vi "Laser Fine Cutting.vi"(0 "configuration file path":path=path "C:/Users/admin/OneDrive/文档/Inlafa.CCV254.MES/System/All Config.ini" caption="配置文件的路径", 1 "fine cutting msic":T1) -> ()   [LabVIEW 2018]
uses:
  Ctl.xio/fine cutting msic ctl.ctl
  SubVIS.xio/DataSocket/DataSocket_Tags.ctl
  Ctl.xio/part type.ctl
  SubVIS.xio/Creat Write List VI's/DefCtrl/Station.ctl
  SubVIS.xio/DataSocket/Write PLC Vars/Write String Var in.vi
  <vilib>/Utility/file.llb/Read From Spreadsheet File (string).vi
  SubVIS.xio/DataSocket/Write PLC Vars/Write Bool Var in.vi
  SubVIS.xio/DataSocket/Read PLC Vars/Read String Var.vi
  SubVIS.xio/DataSocket/Write PLC Vars/Write Dbl Var in.vi
  SubVIS.xio/DataSocket/Read PLC Vars/Read Bool Var.vi
panel:
  in  "SQL information":string
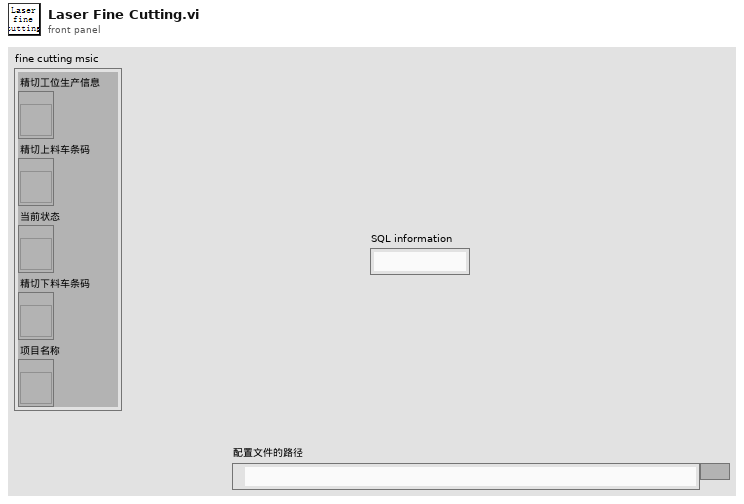
[diagram p1: front panel]
types:
  T1 = cluster{"精切工位生产信息":refnum<vi>, "精切上料车条码":refnum<vi>, "当前状态":refnum<vi>, "精切下料车条码":refnum<vi>, "项目名称":refnum<vi>}
  T2 = typedef "Station.ctl" = enum16{"粗切工位", "热处理工位", "精切工位", "PDF焊接工位", "打凹点预载力工位", "收卷工位", "EOL工位"}
  T3 = typedef "fine cutting msic ctl.ctl" = cluster{"configuration file path":path, "DsOut":T4[], "incar information A":cluster{"incar code":string, "incar No":string, "incar plate No":string, "cut time":string}, "pallet A.No_output":i32, "SQL information":string, "Database":string[], "Serial number":i32, "database path":path, "fine cutting msic":cluster{"production info":refnum<vi>, "incar code":refnum<vi>, "status":refnum<vi>, "outcar code":refnum<vi>, "part type":refnum<vi>}, "part type":T5, "scanner1 coms":string, "scanner2 coms":string, "scanner1 resource name out":refnum<visa-resource-name>, "scanner2 resource name out":refnum<visa-resource-name>, "incar code A":string, "outcar code":string, "outcar information":cluster{"outcar code":string, "outcar No":string, "outcar plate No":string, "cut time":string}, "scanner1 ip ID":refnum<k5>, "scanner2 ip ID":refnum<k5>, "Number of scans":i32, "Cut file":string, "Process code":string, "second?":bool, "incar code B":string, "incar information B":cluster{"incar code":string, "incar No":string, "incar plate No":string, "cut time":string}, "pallet B.No_output":i32}
  T4 = typedef "DataSocket_Tags.ctl" = cluster{"Ds ID":refnum<k13>, "Tag":string}
  T5 = typedef "part type.ctl" = cluster{"Part type":string, "Material code":string, "Part number":string, "Supplier code":string, "Line code":string, "Customer code":string, "Color code":string, "Upper limit":i32, "Temperature":string, "Tot time":string, "EOL stations":string}
  T6 = cluster{"incar code":string, "incar No":string, "incar plate No":string, "cut time":string}
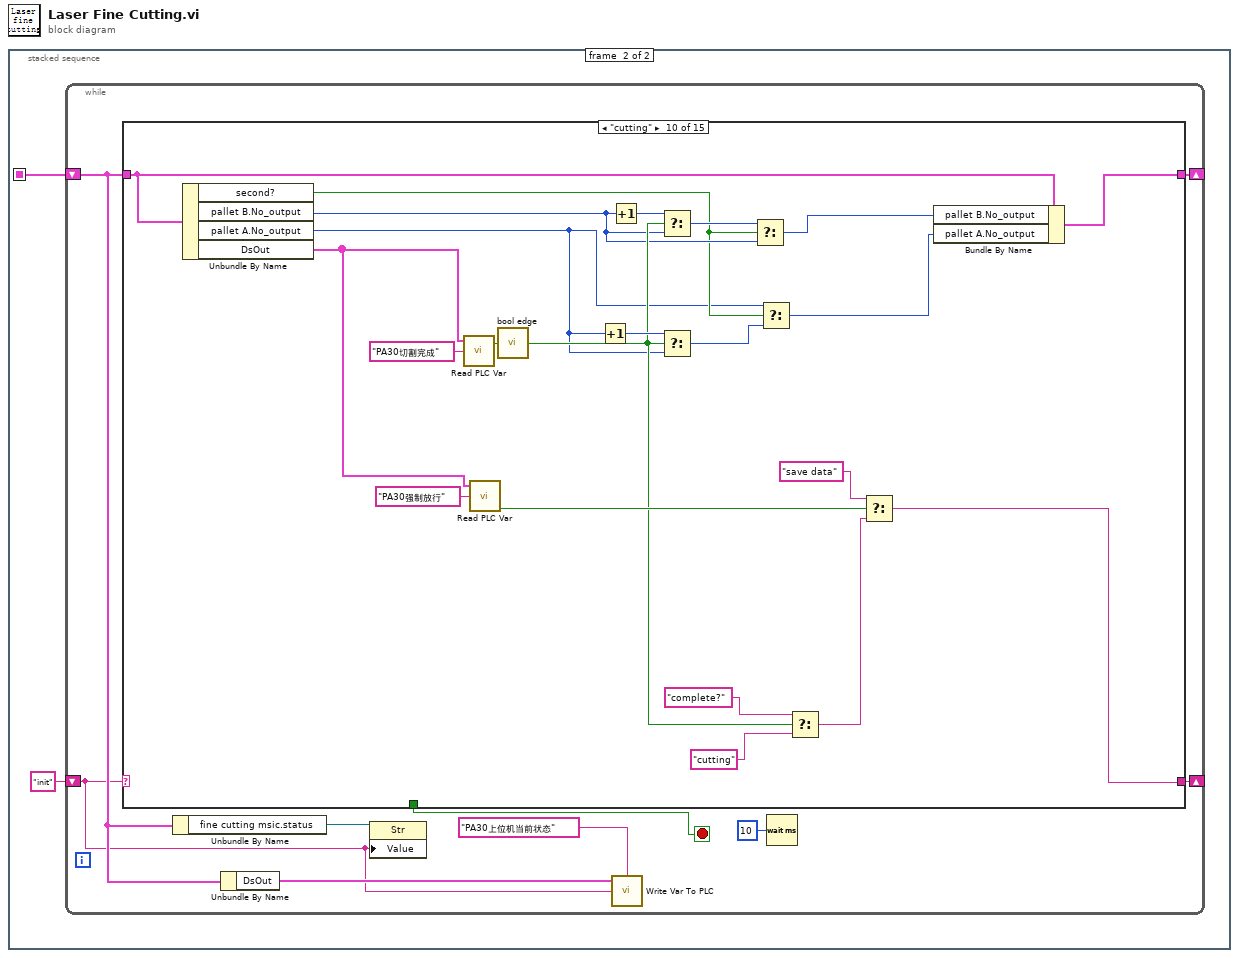
[diagram p0: block diagram]
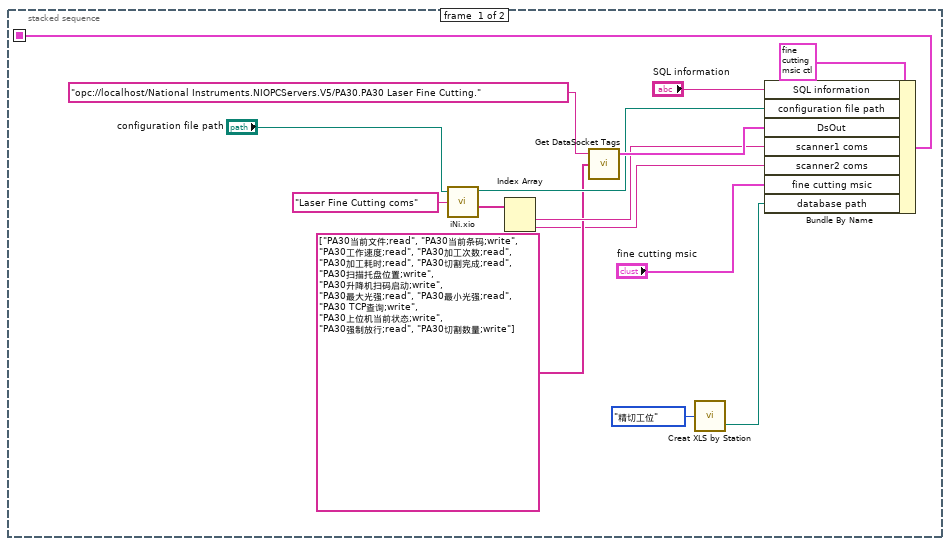
[diagram p2: hidden frame]
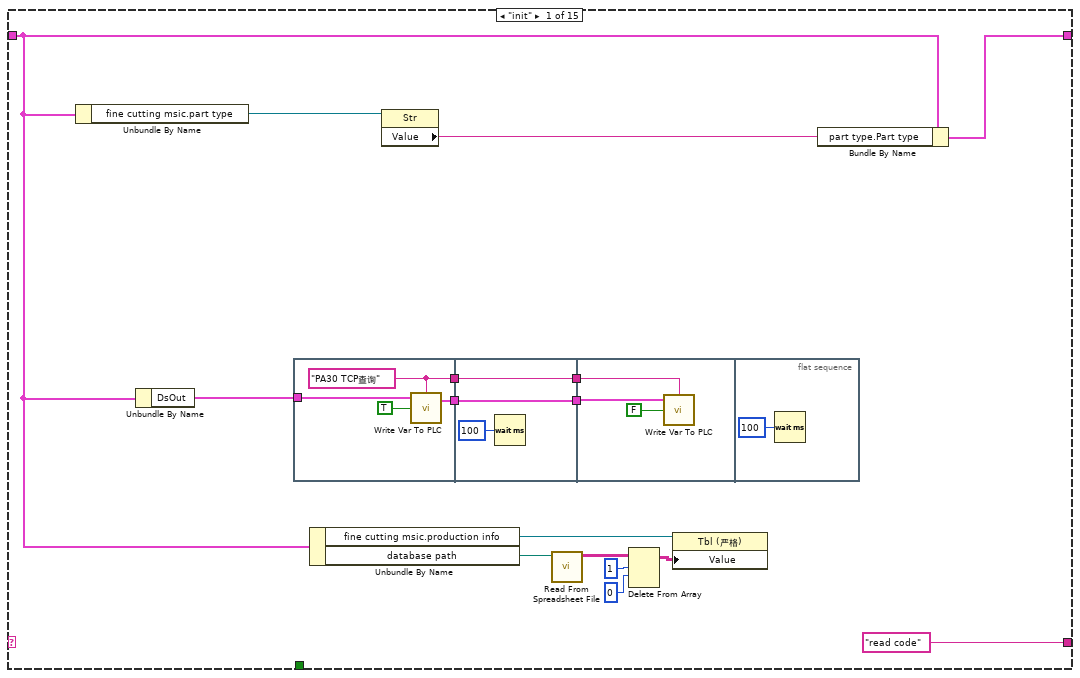
[diagram p3: hidden frame]
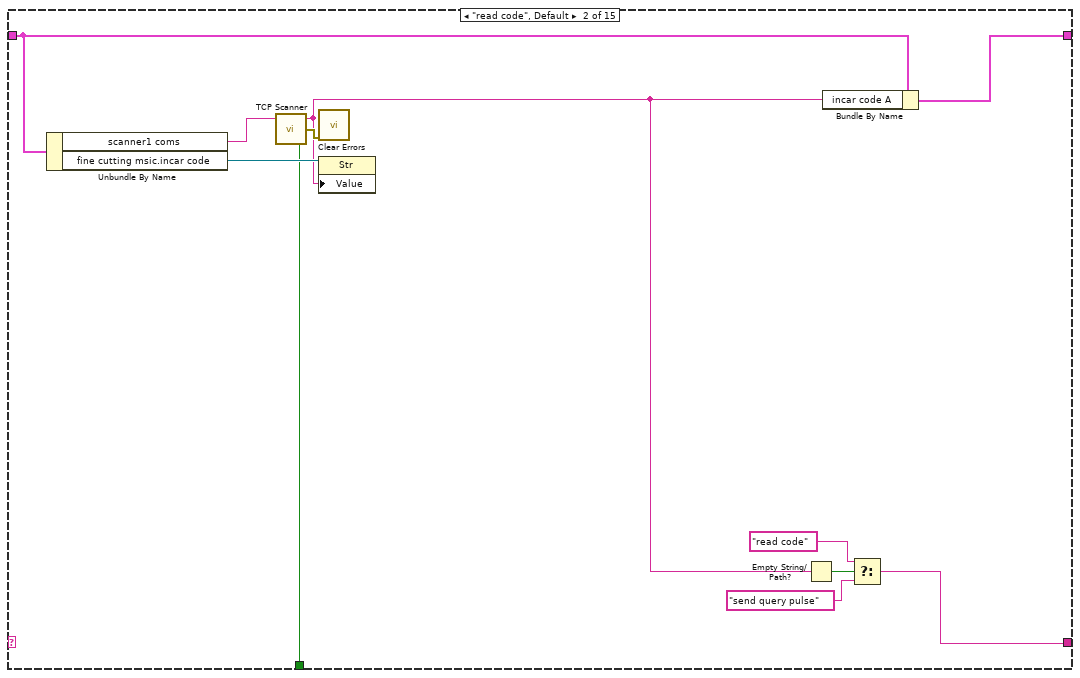
[diagram p4: hidden frame]
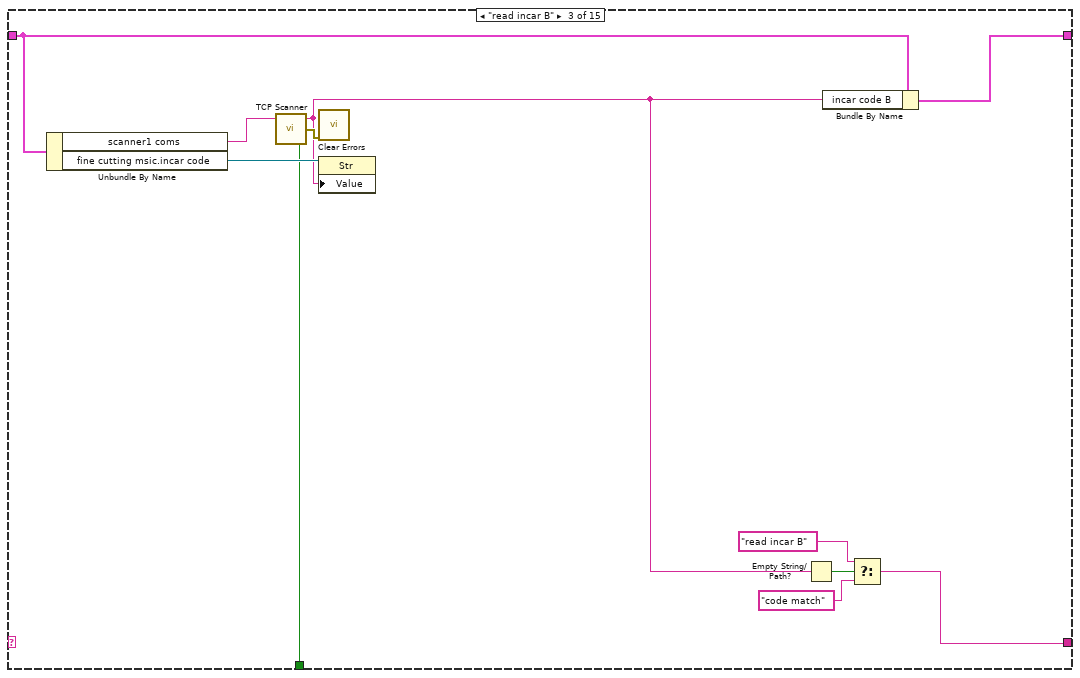
[diagram p5: hidden frame]
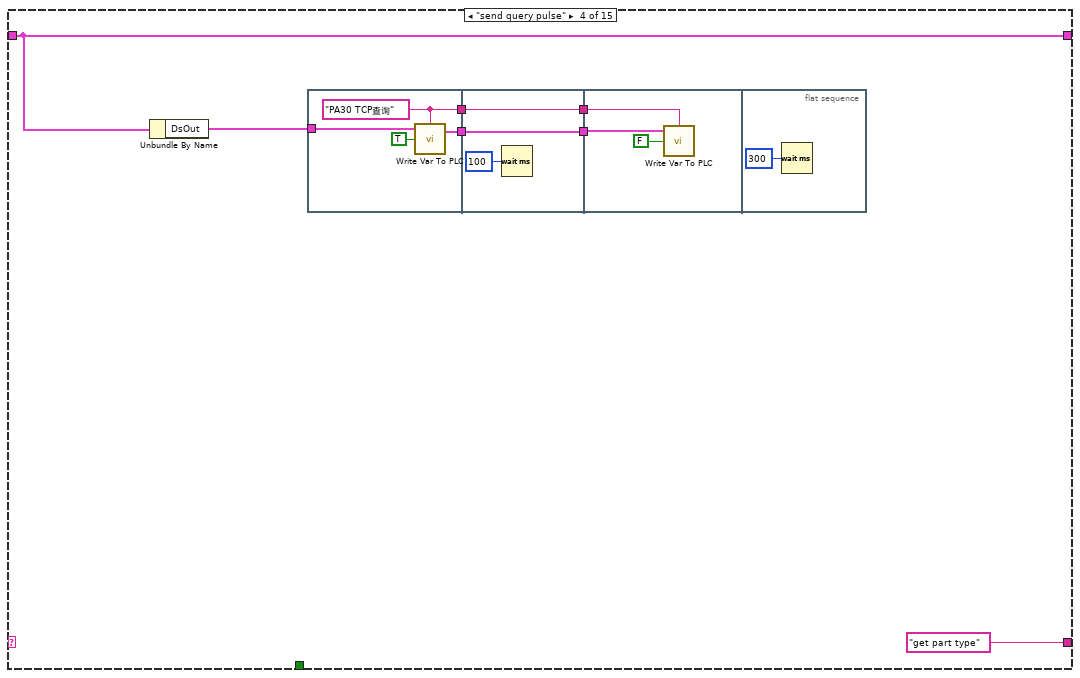
[diagram p6: hidden frame]
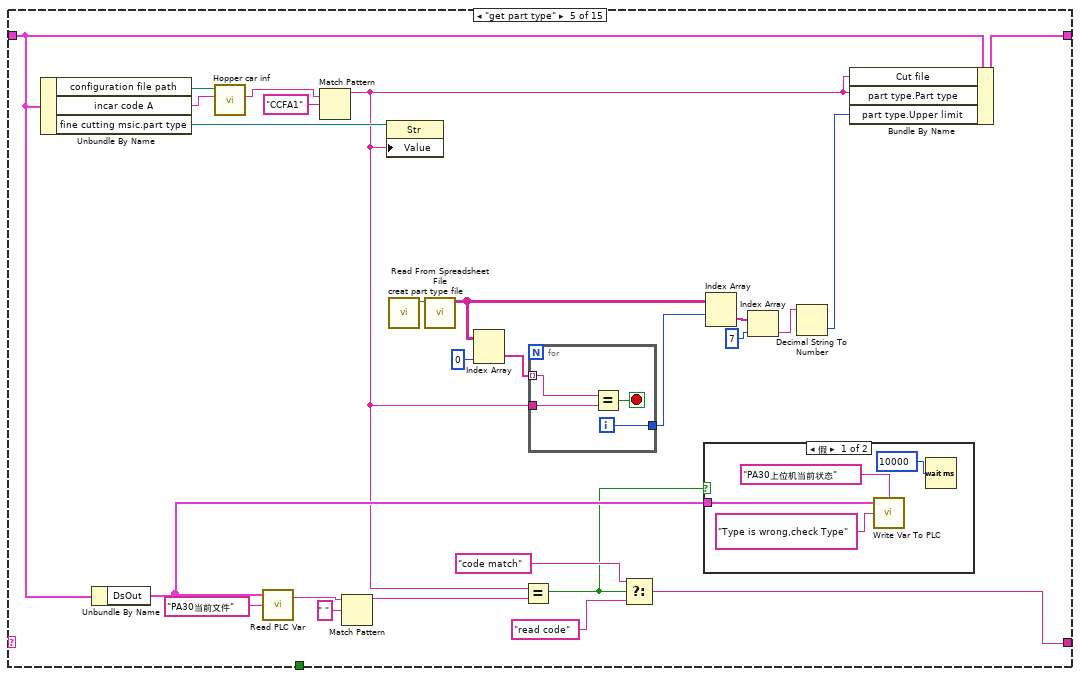
[diagram p7: hidden frame]
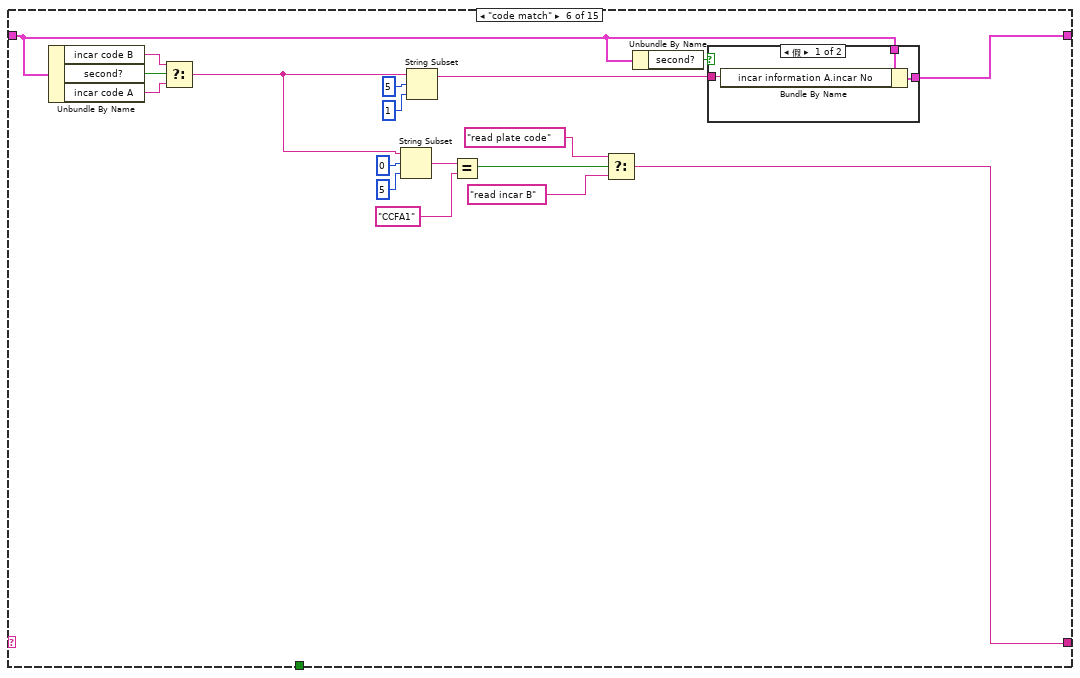
[diagram p9: hidden frame]
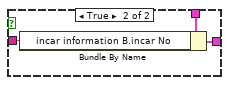
[diagram p10: hidden frame]
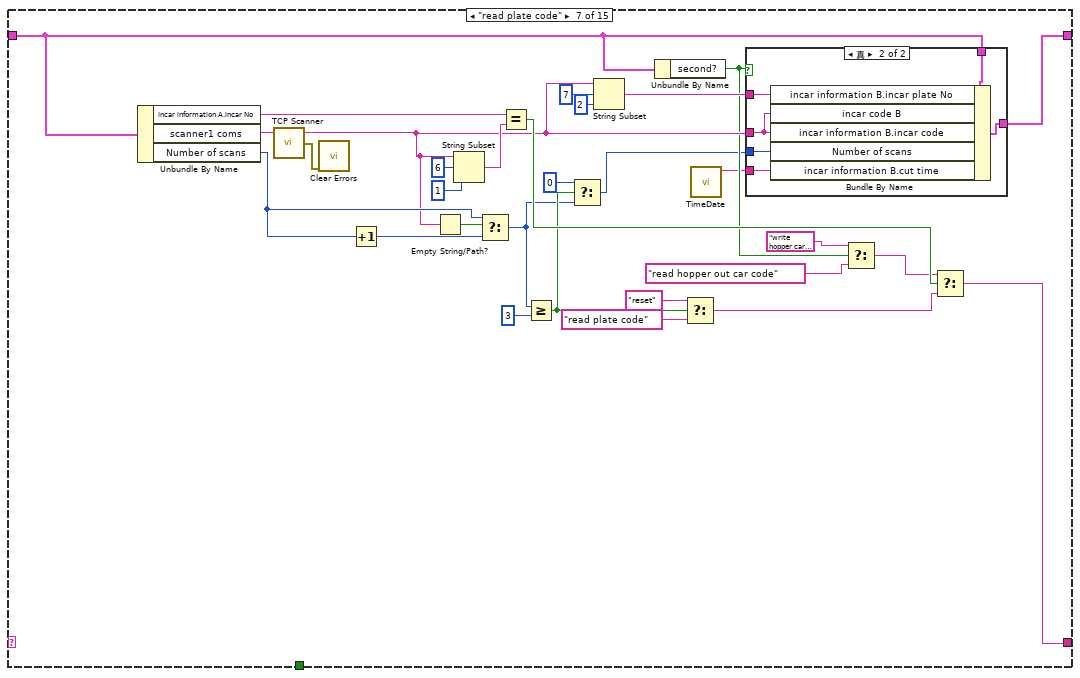
[diagram p11: hidden frame]
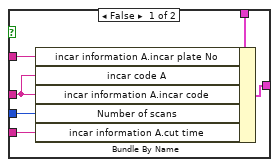
[diagram p12: hidden frame]
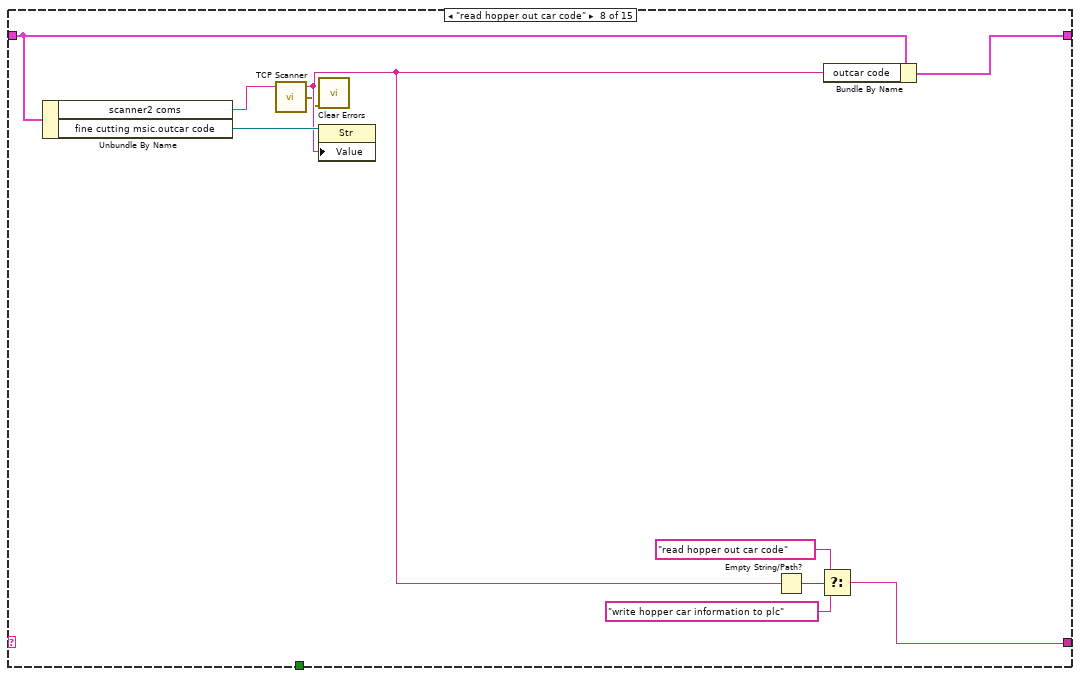
[diagram p13: hidden frame]
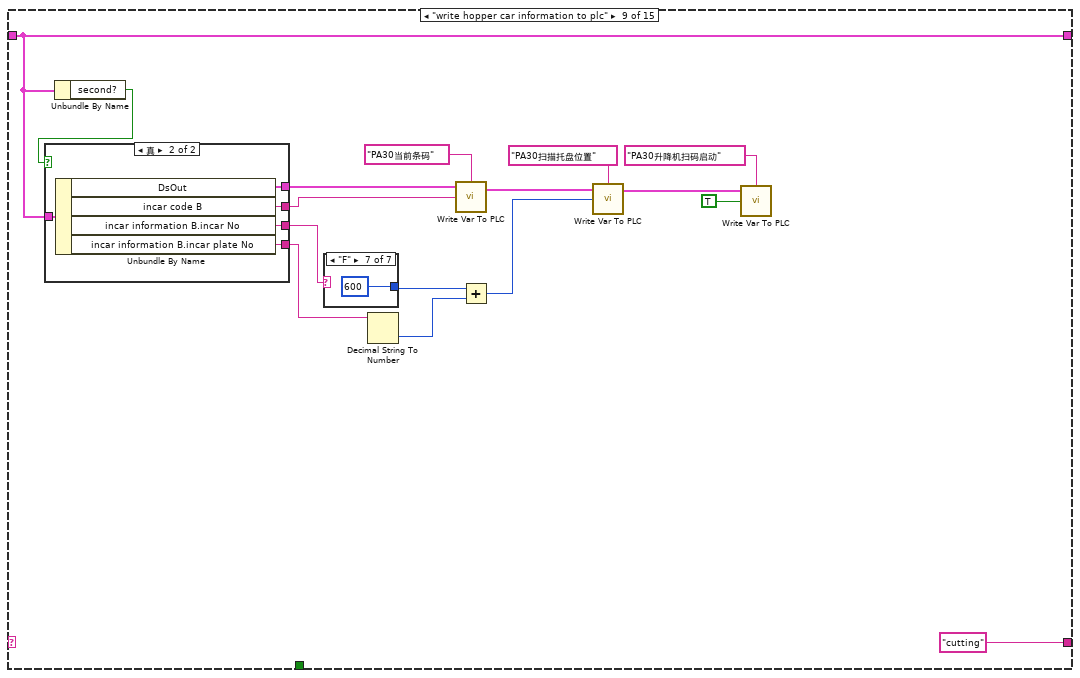
[diagram p14: hidden frame]
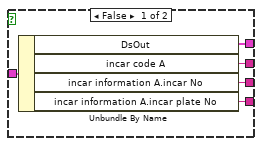
[diagram p15: hidden frame]
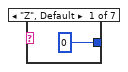
[diagram p16: hidden frame]
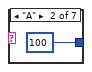
[diagram p17: hidden frame]
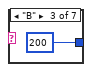
[diagram p18: hidden frame]
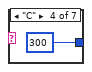
[diagram p19: hidden frame]
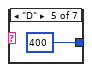
[diagram p20: hidden frame]
diagram:
  n1 = stacked-sequence {
    seq-local: [w3 _] -> [_ w16]
    frame #0 {
      n2 = call "iNi.xio.vi"("configuration file path"="configuration file path", "Sections"="Laser Fine Cutting coms") -> ("configuration file path"=w14:path, "Values"=w12:string[])  [unwired: 1 in, 3 out]
      n3 = Index Array(array=w12) -> (element #1=w11:string, element #2=w5:string)  [unwired: 2 in]
      n4 = call "Get DataSocket Tags.vi"("All Tags"=string[] ["PA30当前文件;read", "PA30当前条码;write", "PA30工作速度;read", "PA30加工次数;read", "PA30加工耗时;read", "PA30切割完成;read", "PA30扫描托盘位置;write", "PA30升降机扫码启动;write", "PA30最大光强;read", "PA30最小光强;read", "PA30 TCP查询;write", "PA30上位机当前状态;write", "PA30强制放行;read", "PA30切割数量;write"], "URL"="opc://localhost/National Instruments.NIOPCServers.V5/PA30.PA30 Laser Fine Cutting.") -> ("DsOut"=w15:T4[])  [unwired: 3 in]
      n5 = call "Creat XLS by Station.vi"("staiton"=Station."精切工位") -> ("new file path (Not A Path if cancelled)"=w2:path)  [unwired: 5 in]
      n6 = Bundle By Name(cluster=T3 {"configuration file path"=path "", "DsOut"=[], "incar information A"={"incar code"="", "incar No"="", "incar plate No"="", "cut time"=""}, "pallet A.No_output"=0, "SQL information"="", "Database"=[], "Serial number"=0, "database path"=path "", "fine cutting msic"={"production info"=refnum, "incar code"=refnum, "status"=refnum, "outcar code"=refnum, "part type"=refnum}, "part type"={"Part type"="", "Material code"="", "Part number"="", "Supplier code"="", "Line code"="", "Customer code"="", "Color code"="", "Upper limit"=0, "Temperature"="", "Tot time"="", "EOL stations"=""}, "scanner1 coms"="", "scanner2 coms"="", "scanner1 resource name out"="", "scanner2 resource name out"="", "incar code A"="", "outcar code"="", "outcar information"={"outcar code"="", "outcar No"="", "outcar plate No"="", "cut time"=""}, "scanner1 ip ID"=refnum, "scanner2 ip ID"=refnum, "Number of scans"=0, "Cut file"="", "Process code"="", "second?"=FALSE, "incar code B"="", "incar information B"={"incar code"="", "incar No"="", "incar plate No"="", "cut time"=""}, "pallet B.No_output"=0} ("rough cutting msic"), "SQL information"="SQL information", "configuration file path"=w14, "DsOut"=w15, "scanner1 coms"=w11, "scanner2 coms"=w5, "fine cutting msic"="fine cutting msic", "database path"=w2) -> (w3:T3)
    }
    frame #1 {
      n7 = while {
        shift-right: [w26] -> _
        shift-left: w16 -> [w21]
        shift-right: [w25] -> _
        shift-left: "init" ("event") -> [w19]
        stop <- w18 stop-if-true
        n8 = case shown="\"cutting\"" w19 {
          tunnel: w21 -> [w27 w62 w73 w77 w101 w129 w161 w201 w206 w256 w263 w287 w302 w309 w320]
          tunnel: [w42 w64 w75 w77 w119 w141 w170 w203 w206 w257 w268 w289 w303 w309 w323] -> w26
          tunnel: ["read code" w56 w67 "get part type" ("f") w100 w139 w171 w196 "cutting" ("event") w246 w267 "database write" ("f") "updata display" ("f") "reset" ("f") "read code" ("f")] -> w25
          tunnel: [_ w54 w65 _ _ _ _ _ _ _ _ _ _ _ _] -> w18
          frame "init" {
            n9 = Unbundle By Name(w27) -> ("fine cutting msic.part type"=w40:refnum<vi>)
            n10 = Unbundle By Name(w27) -> ("DsOut"=w34:T4[])
            n11 = flat-sequence {
              tunnel: w34 -> [w46]
              tunnel: [w44] -> w38
              tunnel: [w43] -> w37
              tunnel: w38 -> [w48]
              tunnel: [w48] -> w36
              tunnel: w37 -> [w47]
              tunnel: [w47] -> w35
              tunnel: w36 -> [w52]
              tunnel: w35 -> [w50]
              frame #0 {
                w43 = "PA30 TCP查询" ("Tag IN")
                n12 = call-poly "Write Var To PLC.vi"("Tag IN"=w43, "Bool Var in"=TRUE, "Ds PLCTags IN"=w46) -> ("Ds PLCTags OUT"=w44:T4[])  [unwired: 1 in, 1 out]
              }
              frame #1 {
                n13 = Wait (ms)(milliseconds to wait=u32 100 ("等待时间（毫秒）")) -> ()  [unwired: 1 out]
              }
              frame #2 {
                n14 = call-poly "Write Var To PLC.vi"("Tag IN"=w50, "Bool Var in"=FALSE, "Ds PLCTags IN"=w52) -> ()  [unwired: 1 in, 2 out]
              }
              frame #3 {
                n15 = Wait (ms)(milliseconds to wait=u32 100 ("等待时间（毫秒）")) -> ()  [unwired: 1 out]
              }
            }
            n16 = Unbundle By Name(w27) -> ("fine cutting msic.production info"=w33:refnum<vi>, "database path"=w32:path)
            n17 = property class="Str"(reference=w40) -> ("Value"=w39:string)  [unwired: 1 in, 2 out]
            n18 = call-poly <vilib>:"Read From Spreadsheet File.vi"("file path (dialog if empty)"=w32) -> ("all rows"=w31:string[][])  [unwired: 6 in, 4 out]
            n19 = Delete From Array(array=w31, length=1 ("长度"), index (row)=0 ("索引 (行)")) -> (array with subset deleted=w28:string[][])  [unwired: 1 in, 1 out]
            n20 = property class="Tbl (严格)"(reference=w33, "Value"=w28) -> ()  [unwired: 1 in, 2 out]
            n21 = Bundle By Name(cluster=w27, "part type.Part type"=w39) -> (w42:T3)
          }
          frame "read code", Default {
            n22 = Unbundle By Name(w62) -> ("scanner1 coms"=w61:string, "fine cutting msic.incar code"=w63:refnum<vi>)
            n23 = call "TCP Scanner.vi"("ip"=w61) -> ("status"=w54:bool, "错误输出"=w60:errorcluster, "Barcode"=w55:string)  [unwired: 2 in]
            n24 = call <vilib>:"Clear Errors.vi"("error in (no error)"=w60) -> ()  [unwired: 5 in, 2 out]
            n25 = property class="Str"(reference=w63, "Value"=w55) -> ()  [unwired: 1 in, 2 out]
            n26 = Empty String/Path?(string/path=w55) -> (empty?=w59:bool)
            n27 = Bundle By Name(cluster=w62, "incar code A"=w55) -> (w64:T3)
            n28 = Select(t="read code", s=w59, f="send query pulse") -> (s? t:f=w56:string)
          }
          frame "read incar B" {
            n29 = Unbundle By Name(w73) -> ("scanner1 coms"=w72:string, "fine cutting msic.incar code"=w74:refnum<vi>)
            n30 = call "TCP Scanner.vi"("ip"=w72) -> ("status"=w65:bool, "错误输出"=w71:errorcluster, "Barcode"=w66:string)  [unwired: 2 in]
            n31 = call <vilib>:"Clear Errors.vi"("error in (no error)"=w71) -> ()  [unwired: 5 in, 2 out]
            n32 = property class="Str"(reference=w74, "Value"=w66) -> ()  [unwired: 1 in, 2 out]
            n33 = Empty String/Path?(string/path=w66) -> (empty?=w70:bool)
            n34 = Bundle By Name(cluster=w73, "incar code B"=w66) -> (w75:T3)
            n35 = Select(t="read incar B", s=w70, f="code match") -> (s? t:f=w67:string)
          }
          frame "send query pulse" {
            n36 = Unbundle By Name(w77) -> ("DsOut"=w78:T4[])
            n37 = flat-sequence {
              tunnel: w78 -> [w86]
              tunnel: [w84] -> w82
              tunnel: [w83] -> w81
              tunnel: w82 -> [w88]
              tunnel: [w88] -> w80
              tunnel: w81 -> [w87]
              tunnel: [w87] -> w79
              tunnel: w80 -> [w92]
              tunnel: w79 -> [w90]
              frame #0 {
                w83 = "PA30 TCP查询" ("Tag IN")
                n38 = call-poly "Write Var To PLC.vi"("Tag IN"=w83, "Bool Var in"=TRUE, "Ds PLCTags IN"=w86) -> ("Ds PLCTags OUT"=w84:T4[])  [unwired: 1 in, 1 out]
              }
              frame #1 {
                n39 = Wait (ms)(milliseconds to wait=u32 100 ("等待时间（毫秒）")) -> ()  [unwired: 1 out]
              }
              frame #2 {
                n40 = call-poly "Write Var To PLC.vi"("Tag IN"=w90, "Bool Var in"=FALSE, "Ds PLCTags IN"=w92) -> ()  [unwired: 1 in, 2 out]
              }
              frame #3 {
                n41 = Wait (ms)(milliseconds to wait=u32 300 ("等待时间（毫秒）")) -> ()  [unwired: 1 out]
              }
            }
          }
          frame "get part type" {
            n42 = Unbundle By Name(w101) -> ("configuration file path"=w109:path, "incar code A"=w108:string, "fine cutting msic.part type"=w107:refnum<vi>)
            n43 = Unbundle By Name(w101) -> ("DsOut"=w96:T4[])
            n44 = call "Hopper car inf.vi"("key"=w108, "path in"=w109) -> ("value out"=w106:string)  [unwired: 8 in, 1 out]
            n45 = call-poly "Read PLC Var.vi"("Tag IN"="PA30当前文件", "Ds PLCTags IN"=w96) -> ("String Var out"=w99:string)  [unwired: 1 in, 1 out]
            n46 = Match Pattern(string=w106, regular expression="CCFA1" ("正则表达式")) -> (before substring=w94:string)  [unwired: 1 in, 3 out]
            n47 = Match Pattern(string=w99, regular expression=" " ("正则表达式")) -> (before substring=w97:string)  [unwired: 1 in, 3 out]
            n48 = property class="Str"(reference=w107, "Value"=w94) -> ()  [unwired: 1 in, 2 out]
            n49 = call "creat part type file.vi"() -> ("new file path (Not A Path if cancelled)"=w110:path)  [unwired: 11 in]
            n50 = call-poly <vilib>:"Read From Spreadsheet File.vi"("file path (dialog if empty)"=w110) -> ("all rows"=w114:string[][])  [unwired: 6 in, 4 out]
            n51 = Index Array(array=w114, index (col)=0 ("禁用的索引 (列)")) -> (element=w115:string[])  [unwired: 1 in]
            n52 = Equal?(x=w94, y=w97) -> (x = y?=w95:bool)
            n53 = for {
              tunnel: w115 -> [w124] mode=indexing
              tunnel: [w126] -> w113
              tunnel: w94 -> [w125]
              i -> [w126]
              stop <- w127 stop-if-true
              n54 = Equal?(x=w124, y=w125) -> (x = y?=w127:bool)
            }
            n55 = Select(t="code match" ("event"), s=w95, f="read code" ("event")) -> (s? t:f=w100:string)
            n56 = case shown="假" w95 {
              tunnel: w96 -> [w123 _]
              frame False {
                n57 = call-poly "Write Var To PLC.vi"("Tag IN"="PA30上位机当前状态", "String Var in"="Type is wrong,check Type", "Ds PLCTags IN"=w123) -> ()  [unwired: 1 in, 2 out]
                n58 = Wait (ms)(milliseconds to wait=u32 10000 ("等待时间（毫秒）")) -> ()  [unwired: 1 out]
              }
              frame True {
              }
            }
            n59 = Index Array(array=w114, index (row)=w113) -> (element=w112:string[])  [unwired: 1 in]
            n60 = Index Array(array=w112, index=7 ("索引")) -> (element=w117:string)
            n61 = Decimal String To Number(string=w117) -> (number=w111:i32)  [unwired: 2 in, 1 out]
            n62 = Bundle By Name(cluster=w101, "Cut file"=w94, "part type.Part type"=w94, "part type.Upper limit"=w111) -> (w119:T3)
          }
          frame "code match" {
            n63 = Unbundle By Name(w129) -> ("incar code B"=w132:string, "second?"=w133:bool, "incar code A"=w130:string)
            n64 = Select(t=w132, s=w133, f=w130) -> (s? t:f=w131:string)
            n65 = String Subset(string=w131, offset (0)=0 ("偏移量(0)"), length (rest)=5 ("长度（剩余）")) -> (substring=w137:string)
            n66 = String Subset(string=w131, offset (0)=5 ("偏移量(0)"), length (rest)=1 ("长度（剩余）")) -> (substring=w136:string)
            n67 = Equal?(x=w137, y="CCFA1") -> (x = y?=w140:bool)
            n68 = Select(t="read plate code" ("event"), s=w140, f="read incar B" ("event")) -> (s? t:f=w139:string)
            n69 = Unbundle By Name(w129) -> ("second?"=w128:bool)
            n70 = case shown="假" w128 {
              tunnel: [w146 w151] -> w141
              tunnel: w136 -> [w148 w150]
              tunnel: w129 -> [w147 w149]
              frame False {
                n71 = Bundle By Name(cluster=w147, "incar information A.incar No"=w148) -> (w146:T3)
              }
              frame True {
                n72 = Bundle By Name(cluster=w149, "incar information B.incar No"=w150) -> (w151:T3)
              }
            }
          }
          frame "read plate code" {
            n73 = Unbundle By Name(w161) -> ("incar information A.incar No"=w178:string, "scanner1 coms"=w181:string, "Number of scans"=w167:i32)
            n74 = call "TCP Scanner.vi"("ip"=w181) -> ("错误输出"=w169:errorcluster, "Barcode"=w162:string)  [unwired: 2 in, 1 out]
            n75 = call <vilib>:"Clear Errors.vi"("error in (no error)"=w169) -> ()  [unwired: 5 in, 2 out]
            n76 = Increment(x=w167) -> (x+1=w166:i32)
            n77 = Empty String/Path?(string/path=w162) -> (empty?=w168:bool)
            n78 = String Subset(string=w162, offset (0)=6 ("偏移量(0)"), length (rest)=1 ("长度（剩余）")) -> (substring=w176:string)
            n79 = Select(t=w167, s=w168, f=w166) -> (s? t:f=w154:i32)
            n80 = Equal?(x=w178, y=w176) -> (x = y?=w177:bool)
            n81 = Greater Or Equal?(x=w154, y=3) -> (x >= y?=w156:bool)
            n82 = Select(t=0, s=w156, f=w154) -> (s? t:f=w153:i32)
            n83 = String Subset(string=w162, offset (0)=7 ("偏移量(0)"), length (rest)=2 ("长度（剩余）")) -> (substring=w163:string)
            n84 = Unbundle By Name(w161) -> ("second?"=w160:bool)
            n85 = Select(t="reset" ("event"), s=w156, f="read plate code" ("event")) -> (s? t:f=w173:string)
            n86 = call "TimeDate.vi"() -> ("time_YMD"=w152:string)  [unwired: 10 in, 1 out]
            n87 = case shown="真" w160 {
              tunnel: w161 -> [w187 w193]
              tunnel: [w186 w189] -> w170
              tunnel: w153 -> [w185 w190]
              tunnel: w163 -> [w184 w192]
              tunnel: w162 -> [w183 w191]
              tunnel: w152 -> [w182 w188]
              frame False {
                n88 = Bundle By Name(cluster=w187, "incar information A.incar plate No"=w184, "incar code A"=w183, "incar information A.incar code"=w183, "Number of scans"=w185, "incar information A.cut time"=w182) -> (w186:T3)
              }
              frame True {
                n89 = Bundle By Name(cluster=w193, "incar information B.incar plate No"=w192, "incar code B"=w191, "incar information B.incar code"=w191, "Number of scans"=w190, "incar information B.cut time"=w188) -> (w189:T3)
              }
            }
            n90 = Select(t="write hopper car information to plc" ("event"), s=w160, f="read hopper out car code" ("event")) -> (s? t:f=w158:string)
            n91 = Select(t=w158, s=w177, f=w173) -> (s? t:f=w171:string)
          }
          frame "read hopper out car code" {
            n92 = Unbundle By Name(w201) -> ("scanner2 coms"=w195:string, "fine cutting msic.outcar code"=w202:refnum<vi>)
            n93 = call "TCP Scanner.vi"("ip"=w195) -> ("错误输出"=w194:errorcluster, "Barcode"=w200:string)  [unwired: 2 in, 1 out]
            n94 = call <vilib>:"Clear Errors.vi"("error in (no error)"=w194) -> ()  [unwired: 5 in, 2 out]
            n95 = property class="Str"(reference=w202, "Value"=w200) -> ()  [unwired: 1 in, 2 out]
            n96 = Empty String/Path?(string/path=w200) -> (empty?=w199:bool)
            n97 = Select(t="read hopper out car code" ("f"), s=w199, f="write hopper car information to plc") -> (s? t:f=w196:string)
            n98 = Bundle By Name(cluster=w201, "outcar code"=w200) -> (w203:T3)
          }
          frame "write hopper car information to plc" {
            n99 = Unbundle By Name(w206) -> ("second?"=w205:bool)
            n100 = case shown="真" w205 {
              tunnel: [w224 w226] -> w219
              tunnel: [w223 w225] -> w218
              tunnel: [w222 w228] -> w209
              tunnel: [w221 w227] -> w208
              tunnel: w206 -> [w220 w229]
              frame False {
                n101 = Unbundle By Name(w220) -> ("DsOut"=w222:T4[], "incar code A"=w221:string, "incar information A.incar No"=w224:string, "incar information A.incar plate No"=w223:string)
              }
              frame True {
                n102 = Unbundle By Name(w229) -> ("DsOut"=w228:T4[], "incar code B"=w227:string, "incar information B.incar No"=w226:string, "incar information B.incar plate No"=w225:string)
              }
            }
            n103 = case shown="\"F\"" w219 {
              tunnel: [0 100 200 300 400 500 600] -> w217
              frame "Z", Default {
              }
              frame "A" {
              }
              frame "B" {
              }
              frame "C" {
              }
              frame "D" {
              }
              frame "E" {
              }
              frame "F" {
              }
            }
            n104 = Decimal String To Number(string=w218) -> (number=w216:i32)  [unwired: 2 in, 1 out]
            n105 = call-poly "Write Var To PLC.vi"("Tag IN"="PA30当前条码", "String Var in"=w208, "Ds PLCTags IN"=w209) -> ("Ds PLCTags OUT"=w210:T4[])  [unwired: 1 in, 1 out]
            n106 = Add(x=w217, y=w216) -> (x+y=w214:i32)
            n107 = call-poly "Write Var To PLC.vi"("Tag IN"="PA30扫描托盘位置", "Dbl Var in"=w214, "Ds PLCTags IN"=w210) -> ("Ds PLCTags OUT"=w213:T4[])  [unwired: 1 in, 1 out]
            n108 = call-poly "Write Var To PLC.vi"("Tag IN"="PA30升降机扫码启动", "Bool Var in"=TRUE, "Ds PLCTags IN"=w213) -> ()  [unwired: 1 in, 2 out]
          }
          frame "cutting" {
            n109 = Unbundle By Name(w256) -> ("second?"=w240:bool, "pallet B.No_output"=w241:i32, "pallet A.No_output"=w239:i32, "DsOut"=w250:T4[])
            n110 = call-poly "Read PLC Var.vi"("Tag IN"="PA30切割完成", "Ds PLCTags IN"=w250) -> ("Bool Var out"=w252:bool)  [unwired: 1 in, 1 out]
            n111 = call-poly "Read PLC Var.vi"("Tag IN"="PA30强制放行", "Ds PLCTags IN"=w250) -> ("Bool Var out"=w249:bool)  [unwired: 1 in, 1 out]
            n112 = call "bool edge.vi"("bool in"=w252) -> ("true-false"=w245:bool)  [unwired: 6 in, 1 out]
            n113 = Increment(x=w239) -> (x+1=w258:i32)
            n114 = Increment(x=w241) -> (x+1=w244:i32)
            n115 = Select(t=w244, s=w245, f=w241) -> (s? t:f=w243:i32)
            n116 = Select(t=w258, s=w245, f=w239) -> (s? t:f=w238:i32)
            n117 = Select(t=w243, s=w240, f=w241) -> (s? t:f=w242:i32)
            n118 = Select(t=w239, s=w240, f=w238) -> (s? t:f=w237:i32)
            n119 = Select(t="complete?" ("event"), s=w245, f="cutting" ("event")) -> (s? t:f=w247:string)
            n120 = Select(t="save data" ("event"), s=w249, f=w247) -> (s? t:f=w246:string)
            n121 = Bundle By Name(cluster=w256, "pallet B.No_output"=w242, "pallet A.No_output"=w237) -> (w257:T3)
          }
          frame "complete?" {
            n122 = Unbundle By Name(w263) -> ("pallet B.No_output"=w262:i32)
            n123 = Unbundle By Name(w263) -> ("pallet A.No_output"=w261:i32, "part type.Upper limit"=w275:i32, "DsOut"=w272:T4[])
            n124 = Unbundle By Name(w263) -> ("second?"=w264:bool)
            n125 = Select(t=w262, s=w264, f=w261) -> (s? t:f=w260:i32)
            n126 = Select(t="save data" ("event"), s=w264, f="read incar B" ("event")) -> (s? t:f=w265:string)
            n127 = Greater Or Equal?(x=w260, y=w275) -> (x >= y?=w259:bool)
            n128 = Multiply(x=w260, y=2) -> (x*y=w269:i32)
            n129 = Select(t=w265, s=w259, f="cutting") -> (s? t:f=w267:string)
            n130 = call-poly "Write Var To PLC.vi"("Tag IN"="PA30切割数量", "Dbl Var in"=w269, "Ds PLCTags IN"=w272) -> ()  [unwired: 1 in, 2 out]
            n131 = case shown="真" w259 {
              tunnel: [w276 w279] -> w268
              tunnel: w263 -> [w276 w278]
              frame False {
              }
              frame True {
                n132 = Bundle By Name(cluster=w278, "second?"=TRUE) -> (w279:T3)
              }
            }
          }
          frame "save data" {
            n133 = Unbundle By Name(w287) -> ("incar code A"=w288:string, "incar information A.cut time"=w285:string, "incar code B"=w284:string, "incar information B.cut time"=w283:string, "Cut file"=w282:string, "part type.Part type"=w281:string, "outcar code"=w280:string)
            n134 = call "TimeDate.vi"() -> ("time_YMD"=w286:string)  [unwired: 10 in, 1 out]
            n135 = Build Array(w286, w288, w285, w284, w283, w282, w281, w280) -> (w290:string[])
            n136 = Bundle By Name(cluster=w287, "Database"=w290) -> (w289:T3)
          }
          frame "database write" {
            n137 = Unbundle By Name(w302) -> ("Database"=w301:string[], "configuration file path"=w300:path, "incar information A.incar code"=w299:string, "outcar code"=w298:string)
            n138 = call "Hopper car inf.vi"("key"=w299, "path in"=w300) -> ("value out"=w297:string, "path out"=w296:path)  [unwired: 8 in]
            n139 = call "Hopper car inf.vi"("write\\read（read)"=enum16{"read", "write"}."write" ("write\\read（read)"), "value"=w297, "key"=w298, "path in"=w296) -> ()  [unwired: 6 in, 2 out]
            n140 = Build Array (concatenate)(w301, w297) -> (w293:string[])
            n141 = call "Creat XLS by Station.vi"("staiton"=Station."精切工位", "data in"=w293) -> ("new file path (Not A Path if cancelled)"=w294:path)  [unwired: 4 in]
            n142 = Bundle By Name(cluster=w302, "database path"=w294) -> (w303:T3)
          }
          frame "updata display" {
            n143 = Unbundle By Name(w309) -> ("fine cutting msic.production info"=w311:refnum<vi>, "database path"=w310:path)
            n144 = call-poly <vilib>:"Read From Spreadsheet File.vi"("file path (dialog if empty)"=w310) -> ("all rows"=w308:string[][])  [unwired: 6 in, 4 out]
            n145 = Delete From Array(array=w308, length=1 ("长度"), index (row)=0 ("索引 (行)")) -> (array with subset deleted=w305:string[][])  [unwired: 1 in, 1 out]
            n146 = property class="Tbl (严格)"(reference=w311, "Value"=w305) -> ()  [unwired: 1 in, 2 out]
          }
          frame "reset" {
            w314 = T6 {"incar code"="", "incar No"="", "incar plate No"="", "cut time"=""} ("incar information A")
            w313 = 0 ("Number of scans")
            w317 = ""
            w316 = "" ("BarCode")
            n147 = Unbundle By Name(w320) -> ("fine cutting msic.incar code"=w319:refnum<vi>, "fine cutting msic.outcar code"=w318:refnum<vi>)
            n148 = property class="Str"(reference=w319, "Value"=w317) -> ()  [unwired: 1 in, 2 out]
            n149 = property class="Str"(reference=w318, "Value"=w317) -> ()  [unwired: 1 in, 2 out]
            n150 = Bundle By Name(cluster=w320, "pallet B.No_output"=w313, "Number of scans"=w313, "pallet A.No_output"=w313, "incar code A"=w316, "incar code B"=w316, "outcar code"=w316, "Database"=string[] [], "incar information A"=w314, "incar information B"=w314, "outcar information"=w314, "second?"=FALSE) -> (w323:T3)
          }
        }
        n151 = Unbundle By Name(w21) -> ("fine cutting msic.status"=w23:refnum<vi>)
        n152 = Unbundle By Name(w21) -> ("DsOut"=w20:T4[])
        n153 = property class="Str"(reference=w23, "Value"=w19) -> ()  [unwired: 1 in, 2 out]
        n154 = call-poly "Write Var To PLC.vi"("Tag IN"="PA30上位机当前状态", "String Var in"=w19, "Ds PLCTags IN"=w20) -> ()  [unwired: 1 in, 2 out]
        n155 = Wait (ms)(milliseconds to wait=u32 10 ("等待时间（毫秒）")) -> ()  [unwired: 1 out]
      }
    }
  }
